vi "Exsample Grid Cluster.vi"() -> (2 "ref.条件クラスタ":refnum<vi>)   [LabVIEW 2014]
uses:
  Exsample Grid Cluster.ctl
panel:
  in  "条件クラスタ":T1={"選択(列挙体)"=enum."", "数値入力"=0.0, "文字入力"="", "数値入力 2"=100.0, "リング"=0, "ブール"=FALSE, "時間"=0.0} {"時間" format="%<%H:%M:%S.%1u>t"; "リング" items=["リング0"=0, "りんぐ2"=2, "りんぐ255"=255]; "数値入力 2" min=100.0 max=200.0 step=1.0 format="%.1f"; "数値入力" min=0.0 max=1000.0 step=2.0 format="%.1f"}
  # "指定タイプ定義なら、大元のタイプ定義を変更すれば反映される。\n通常のタイプ定義なら、画面で使用しているリファレンスの元の\nクラスタのプロパティで書式変更すること。"
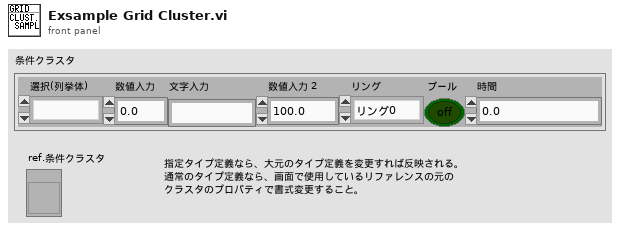
[diagram p1: front panel]
types:
  T1 = typedef "Exsample Grid Cluster.ctl" = cluster{"選択(列挙体)":enum16{"", "STEP2", "RAMP", "aaa"}, "数値入力":dbl, "文字入力":string, "数値入力 2":dbl, "リング":u16, "ブール":bool, "時間":dbl}
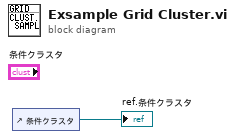
[diagram p0: block diagram]
diagram:
  n1 = control-ref of="条件クラスタ"() -> (→"ref.条件クラスタ":refnum<vi>)
